vi "generate table.vi"(7 "tag select":refnum<vi>, 8 "error in":errorcluster, 9 "DataGridView in":refnum<class "DataGridView.lvclass">, 11 "object ref in":T1) -> (0 "error out":errorcluster, 1 "DataGridView out":refnum<class "DataGridView.lvclass">, 3 "object ref out":T1)   [LabVIEW 2013, in "tag select module editor node.lvclass"]
uses:
  tag select module editor node.lvclass
  LabVIEWdotNetDataGrid/source/DataGridView/DataGridView.lvclass
  object ref.ctl
  <vilib>/NI/Tag Bus Data Framework/Configuration Editor/Classes/Engine Parent/Engine Parent Editor Node.lvclass
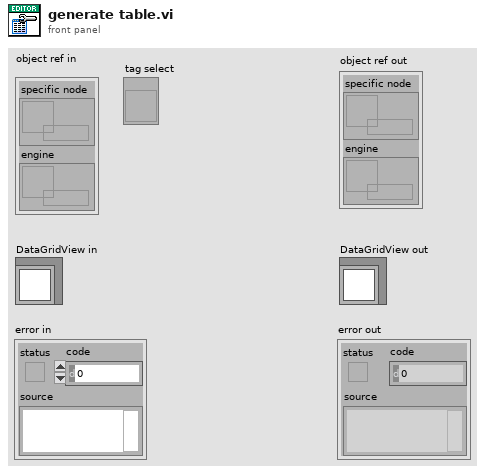
[diagram p1: front panel]
types:
  T1 = typedef "tag select module editor node.lvclass/object ref.ctl" = cluster{"specific node":refnum<data-value>, "engine":refnum<data-value>}
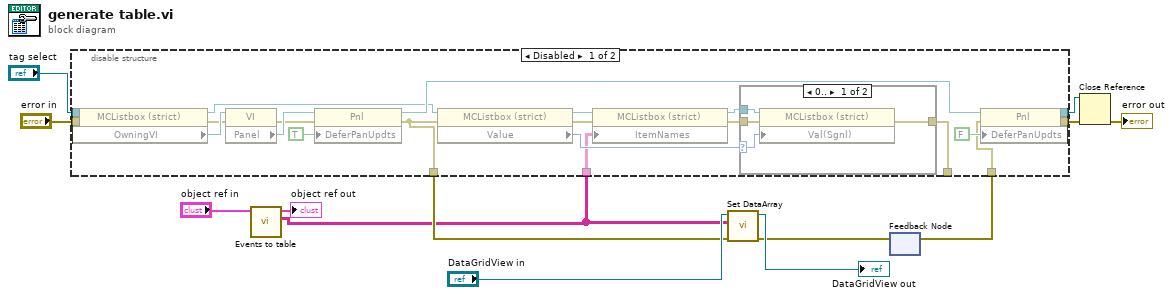
[diagram p0: block diagram]
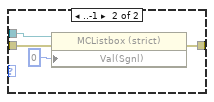
[diagram p2: hidden frame]
diagram:
  n1 = call "Events to table.vi"("object ref in"="object ref in") -> ("table"=w3:string[][], "object ref out"=→"object ref out":T1)  [unwired: 8 in, 1 out]
  n2 = feedback #1() -> (w1:errorcluster)  [unwired: 1 in]
  n3 = disable-structure shown="Disabled" {
    disable-tunnel: [w29 w43] -> w13
    disable-tunnel: "error in" -> [w27 w43]
    disable-tunnel: [w24 _] -> w10
    disable-tunnel: "tag select" -> [w20 _]
    disable-tunnel: [w17 _] -> _
    disable-tunnel: w1 -> [w16 _]
    disable-tunnel: [w15 w43] -> w6
    disable-tunnel: w3 -> [w14 _]
    frame Disabled {
      n4 = property class="MCListbox (strict)"(reference=w20, error in=w27) -> (reference out=w28:refnum<vi>, error out=w25:errorcluster, "OwningVI"=w26:refnum<vi>)
      n5 = property class="VI"(reference=w26, error in=w25) -> (error out=w32:errorcluster, "Panel"=w33:refnum<vi>)  [unwired: 1 out]
      n6 = property class="Pnl"(reference=w33, error in=w32, "DeferPanUpdts"=TRUE ("Defer Panel Updates")) -> (reference out=w30:refnum<vi>, error out=w15:errorcluster)
      n7 = property class="MCListbox (strict)"(reference=w28, error in=w15) -> (reference out=w23:refnum<vi>, error out=w18:errorcluster, "Value"=w19:i32)
      n8 = property class="MCListbox (strict)"(reference=w23, error in=w18, "ItemNames"=w14) -> (reference out=w22:refnum<vi>, error out=w21:errorcluster)
      n9 = case shown="0.." w19 {
        selector: w19 -> [w35 _]
        tunnel: w22 -> [w38 w42]
        tunnel: w21 -> [w37 w41]
        tunnel: [w36 w40] -> w17
        frame 0.. {
          n10 = property class="MCListbox (strict)"(reference=w38, error in=w37, "Val(Sgnl)"=w35) -> (error out=w36:errorcluster)  [unwired: 1 out]
        }
        frame ..-1 {
          n11 = property class="MCListbox (strict)"(reference=w42, error in=w41, "Val(Sgnl)"=0 ("Value (Signaling)")) -> (error out=w40:errorcluster)  [unwired: 1 out]
        }
      }
      n12 = property class="Pnl"(reference=w30, error in=w16, "DeferPanUpdts"=FALSE ("Defer Panel Updates")) -> (reference out=w24:refnum<vi>, error out=w29:errorcluster)
    }
    frame Enabled {
    }
  }
  n13 = call "Set DataArray.vi"("error in"=w6, "Data"=w3, "DataGridView in"="DataGridView in") -> ("error out"=w2:errorcluster, "DataGridView out"=→"DataGridView out":refnum<class "DataGridView.lvclass">)  [unwired: 7 in]
  n14 = feedback-in #1(w2) -> ()
  n15 = Close Reference(reference=w10, error in (no error)=w13) -> (error out=→"error out":errorcluster)
